vi "Get User Interface VI.vi"(8 "error in (no error)":errorcluster, 11 "Thread User Interface in":refnum<class "Thread User Interface.lvclass">) -> (0 "error out":errorcluster, 2 "user interface vi":refnum<vi>, 3 "Thread User Interface out":refnum<class "Thread User Interface.lvclass">)   [LabVIEW 2017, in "PXImc.lvlib" / "Thread User Interface.lvclass"]
uses:
  Thread User Interface.lvclass
  User Interface.vi
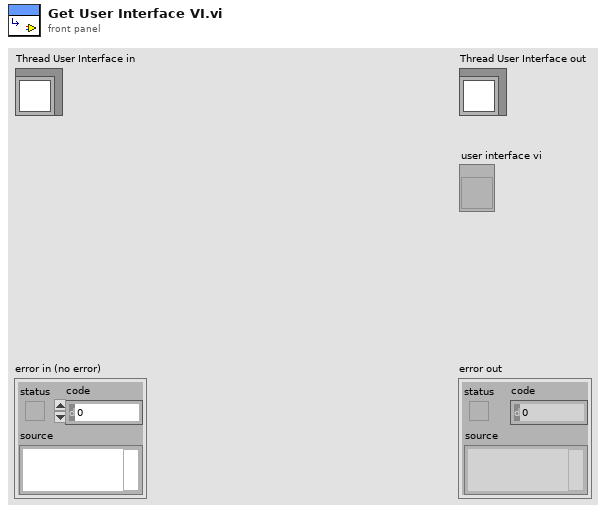
[diagram p1: front panel]
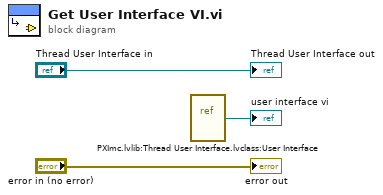
[diagram p0: block diagram]
diagram:
  n1 = vi-ref "PXImc.lvlib:Thread User Interface.lvclass:User Interface.vi"() -> (→"user interface vi":refnum<vi>)
  "error out" <- "error in (no error)"
  "Thread User Interface out" <- "Thread User Interface in"
